vi "calc work.vi"(6 "RL index":i32, 9 "Contact Point index":i32, 10 "X":dbl[](array[numeric]), 11 "Y":dbl[](array[numeric])) -> (2 "area of work":cluster{"Y":dbl[], "Y":dbl[]}[](graph), 3 "WORK":dbl)   [LabVIEW 2015]
uses:
  <vilib>/Analysis/NI_AALPro.lvlib
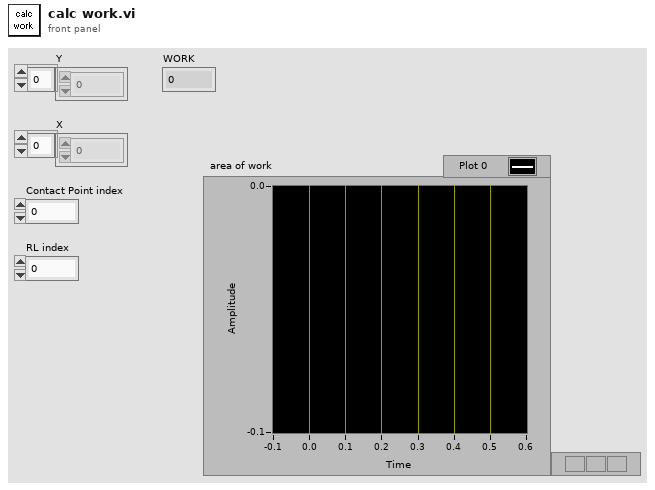
[diagram p1: front panel]
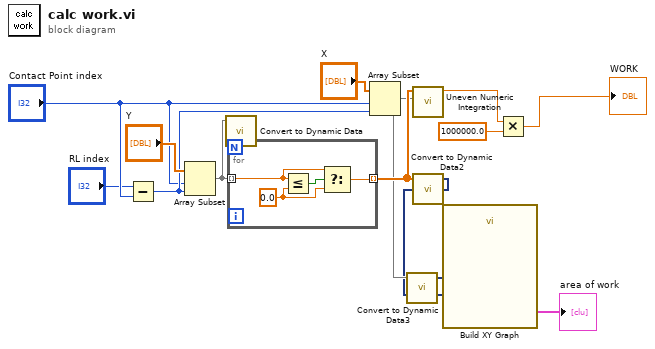
[diagram p0: block diagram]
diagram:
  n1 = Subtract(x="RL index", y="Contact Point index") -> (x-y=w12:i32)
  n2 = Array Subset(array="Y", index="Contact Point index", length=w12) -> (w9:dbl[])
  n3 = call "Convert to Dynamic Data"("Array"=w9) -> ()  [unwired: 3 in, 1 out]
  n4 = for {
    tunnel: w9 -> [w17] mode=indexing
    tunnel: [w15] -> w8 mode=indexing
    w16 = 0.0 ("y")
    n5 = Less Or Equal?(x=w17, y=w16) -> (x <= y?=w18:bool)
    n6 = Select(t=w17, s=w18, f=w16) -> (s? t:f=w15:dbl)
  }
  n7 = Array Subset(array="X", index="Contact Point index", length=w12) -> (w6:dbl[])
  n8 = call "Convert to Dynamic Data3"("Array"=w6) -> ("Dynamic Data Type"=w5:dynamicdata)  [unwired: 3 in]
  n9 = call <vilib>:"Uneven Numeric Integration.vi"("T"=w6, "X"=w8) -> ("result"=w3:dbl)  [unwired: 8 in, 1 out]
  n10 = call "Convert to Dynamic Data2"("Array"=w8) -> ("Dynamic Data Type"=w4:dynamicdata)  [unwired: 3 in]
  n11 = call "Build XY Graph"("Y Input"=w4, "X Input"=w5) -> ("XY Graph"=→"area of work":cluster{"X":dbl[], "Y":dbl[]}[])  [unwired: 8 in, 1 out]
  n12 = Multiply(x=w3, y=1000000.0) -> (x*y=→"WORK":dbl)
